vi "BioFeedback14(Small Buckets +Envelope).vi"(7 "Frames Per Second":dbl=30.0, 9 "Start Trial":bool, 11 "End Trial":bool, 12 "Data Directory":path, 13 "File Name":string, 14 "Extension":string="_EMG.txt") -> ()   [LabVIEW 2016]
uses:
  <vilib>/Waveform/WDTOps.llb/WDT Append Waveforms DBL.vi
  <vilib>/Utility/error.llb/DialogType.ctl
  <vilib>/Utility/file.llb/Write Delimited Spreadsheet (string).vi
  <vilib>/Waveform/WDTFileIO.llb/Export Waveforms To Spreadsheet File (1D).vi
  customSubVIs/Control 1.ctl
panel:
  out "FilteredTrialData One Channel":waveform(dbl)(graph)
  out "Raw Trial Data One  Channel":waveform(dbl)(graph)
  out "DisplayMaxTrialsArray":dbl[][](array[numeric])
  out "DisplayMaxArray":dbl[](array[numeric])
  out "EndProcessTic":u32
  out "StartProcessTic":u32
  out "EndRecordTic":u32
  out "startRecordTic":u32
  out "Start UI":timestamp
  out "UI Elapsed Time":u32
  out "End UI":timestamp
  out "End Process":timestamp
  out "Start Process":timestamp
  out "End Record":timestamp
  out "Start Record":timestamp
  out "Process Elapsed Time":u32
  out "Record Elapsed Time":u32
  out "FilteredTrialData":waveform(dbl)[](graph)
  out "FilteredAndRectified":waveform(dbl)[](graph) caption="Filtered and Rectified"
  out "FilteredTrialData":waveform(dbl)[](array[waveform])
  in  "DisplayChannel":dbl
  out "DisplayTrialData":T1
  out "DisplayValueByChannel":dbl[](array[numeric])
  out "DataBufferSize":dbl
  in  "Big Window Length (s)":dbl=0.5
  out "CurrentAvgByChannel":dbl[](array[numeric])
  out "BigBucketBuilder":dbl[][](array[numeric])
  out "Trial Data Column Headers":string[](array[string])
  in  "TrialDataRowHeaders":string[](array[string])=["Wfm1", "Wfm2", "Wfm3", "Wfm4", "Wfm5", "Wfm6", "Wfm7", "Wfm8"]
  out "GetMaxStartTime":timestamp
  in  "SecondsToAcquireMax":dbl=10.0
  in  "NumberOfMaximumsToTake":dbl=3.0
  in  "CurrentMaxIndex":dbl
  out "SignalsMaxArray":dbl[](array[numeric])
  out "SignalMaxTrialsArray":dbl[][](array[numeric])
  in  "%StdDevIndex":dbl=5.0
  in  "Mean%Index":dbl=4.0
  in  "StdDevIndex":dbl=3.0
  in  "MeanIndex":dbl=2.0
  in  "MaxIndex":dbl=1.0
  in  "MinIndex":dbl
  out "Stability Data":dbl[][](array[numeric])
  out "RawTrialData":waveform(dbl)[](array[waveform])
  in  "UI Ampl Error Path":path=path "C:/Users/Tinggroup/Desktop/VRMuscleActivationVisualizer/VRBiofeedback_v2/assets/BiofeedbackAmplitudeError.txt"
  out "DisplayActivation":dbl
  out "Acquiring Max":bool
  in  "resetMax":bool
  in  "startGetMax":bool
  in  "Amplitude Error":dbl
  in  "UI Data Path":path=path "C:/Users/Tinggroup/Desktop/VRMuscleActivationVisualizer/VRBiofeedback_v2/assets/LeftEMGData.txt"
  in  "EMG Input Device\nProduct Type":string="USB-6009"
  out "DisplayBarActivation":dbl(slide) caption="Left" max=1.0 scale=0.0..100.0
  out "NormalizedSignal8":dbl[](graph)
  out "NormalizedSignal7":dbl[](graph)
  out "NormalizedSignal6":dbl[](graph)
  out "NormalizedSignal5":dbl[](graph)
  out "NormalizedSignal4":dbl[](graph)
  out "NormalizedSignal3":dbl[](graph)
  out "NormalizedSignal2":dbl[](graph)
  out "NormalizedSignal1":dbl[](graph)
  out "Raw Trial Data Wfm":waveform(dbl)[](graph)
  in  "UI Percent Path":path=path "C:/Users/Tinggroup/Desktop/VRMuscleActivationVisualizer/VRBiofeedback_v2/assets/BiofeedbackTargetPercentage.txt"
  in  "Target Percentage":dbl=10.0
  out "Trial In Progress":bool
  in  "Lower Cut-Off":dbl=20.0
  in  "Upper Cut-Off":dbl=300.0
  out "raw data":dynamicdata(graph)
  out "DataBufferIndices":dbl[](array[numeric])
  out "SmallBucketSize":dbl
  out "Samples per frame":dbl
  out "Reset Data Acquisition\nAnd UI Updating":bool=TRUE
  in  "Small Window Length (s)":dbl=0.02
  in  "Sample rate (Hz)":dbl=2000.0
  in  "End Program":bool
  # "Data To Be Saved (Not including Max Data)"
  # "Performance Metrics"
  # "Saving Trial Data"
  # "Small Window"
  # "Set Target"
  # "Scale Max"
  # "Filter and Process Parameters"
  # "MVC Scaling Variables"
  # "Start and end recording for max?"
  # "Big Window"
  # "Display Parameters"
  # "Changes are made instantly and cause moving average to reset to zero"
  # "Analyze Stability of Displayed Data (Not Functional)"
  # "Auto Analyze Stability begins calculating stability\nAs soon as dot enters the target zone and stops \nonce the dot leaves the target zone (Not Yet Implemented)"
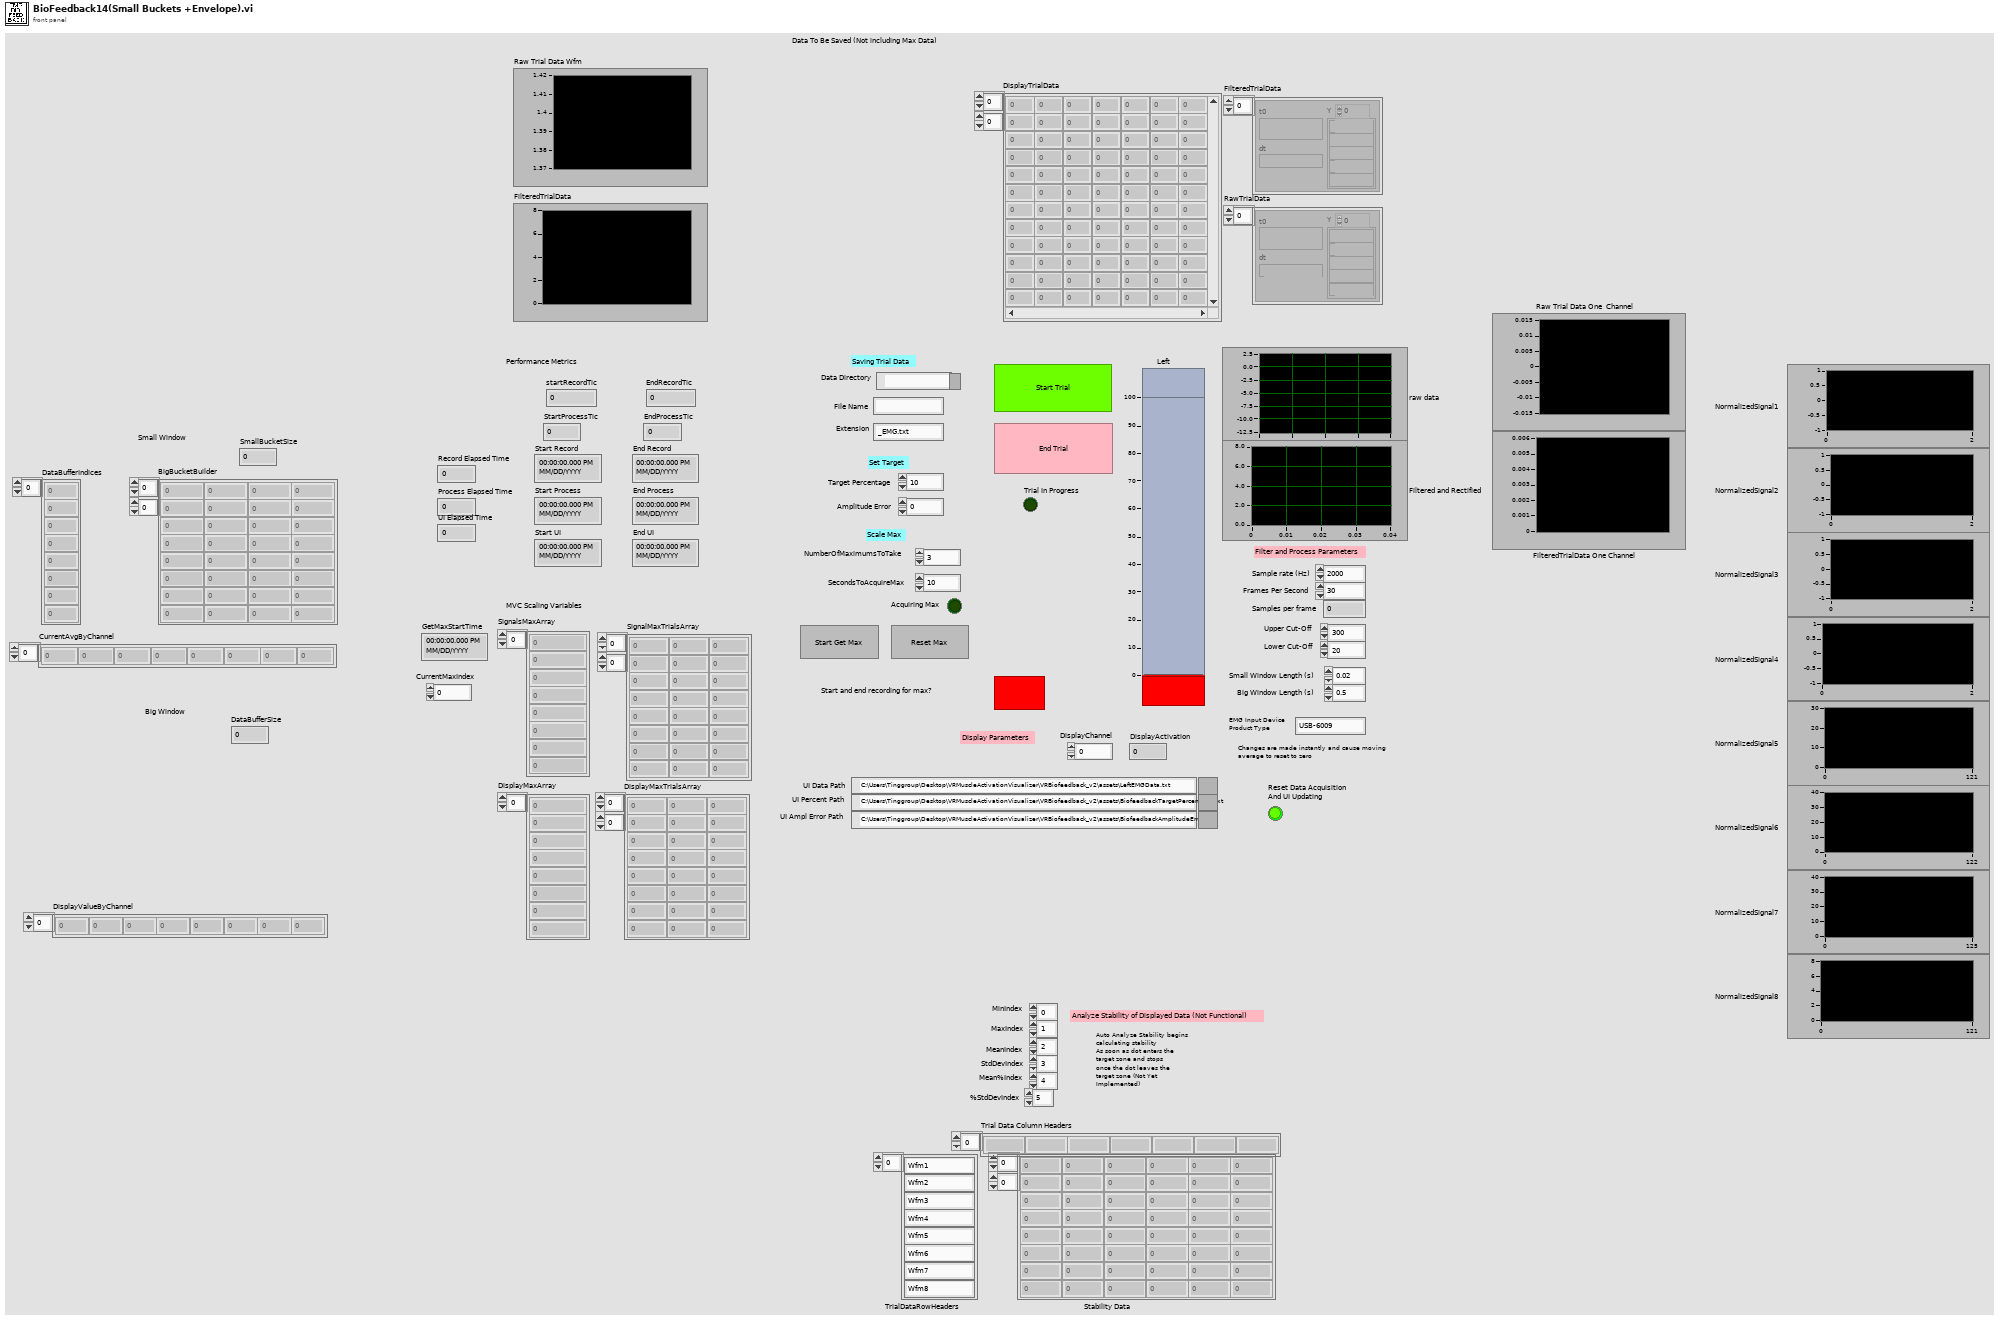
[diagram p1: front panel]
types:
  T1 = typedef "Control 1.ctl" = dbl[][]
  T2 = typedef "DialogType.ctl" = u16
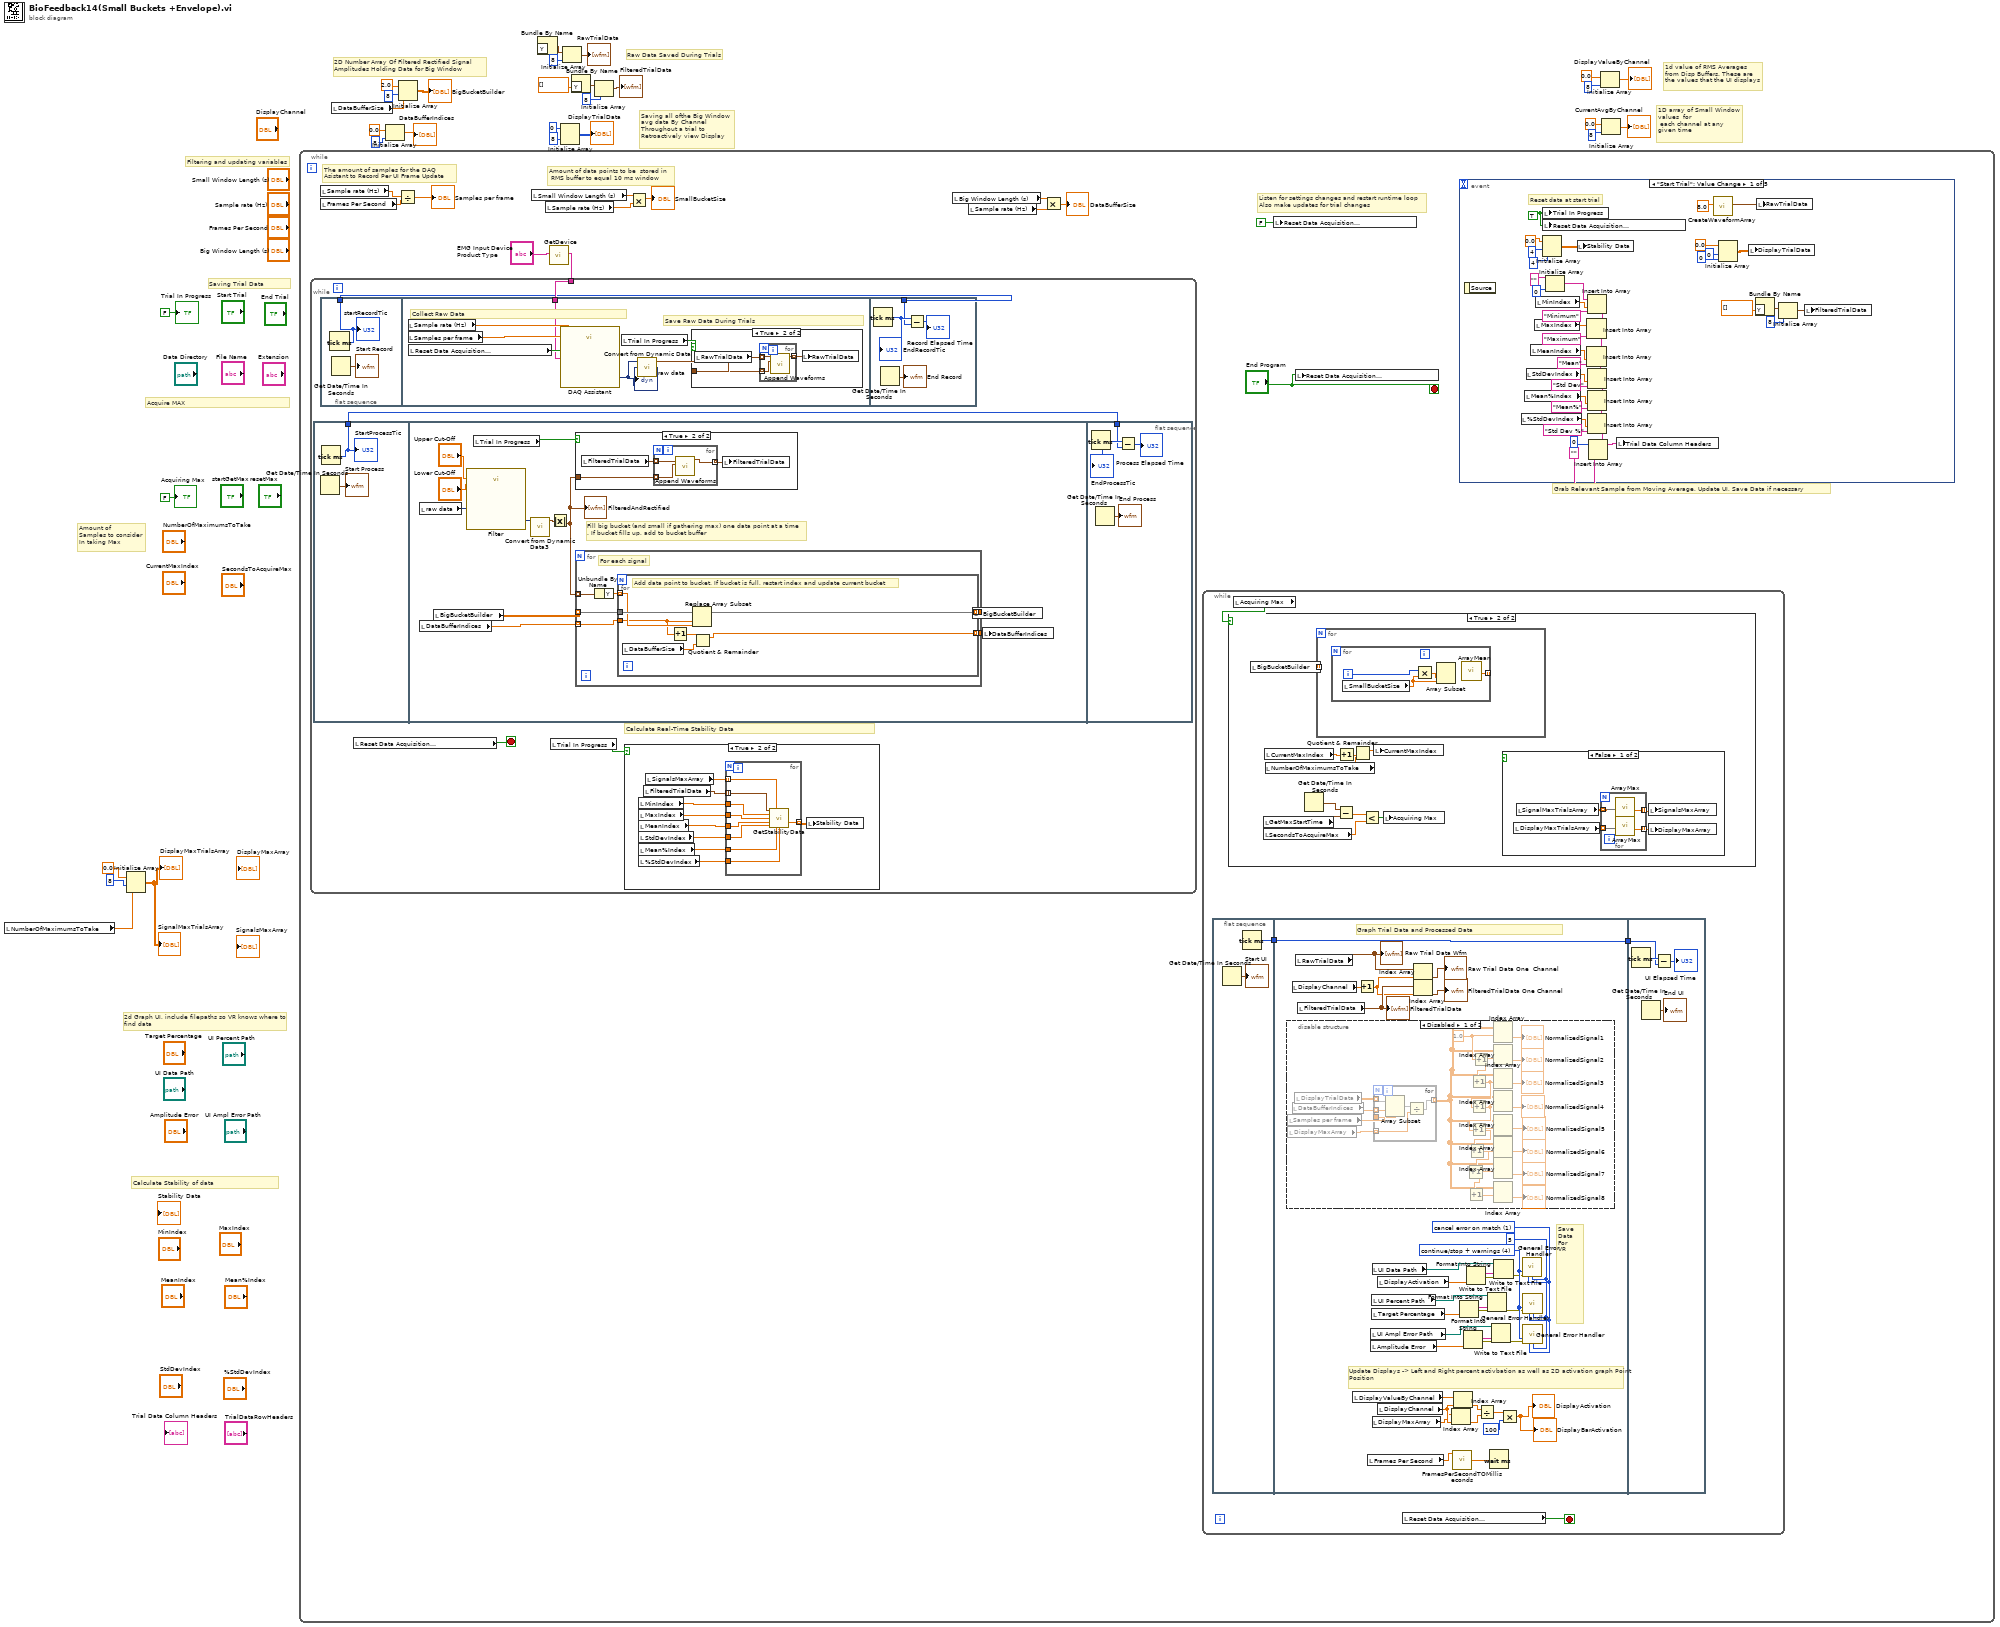
[diagram p0: block diagram]
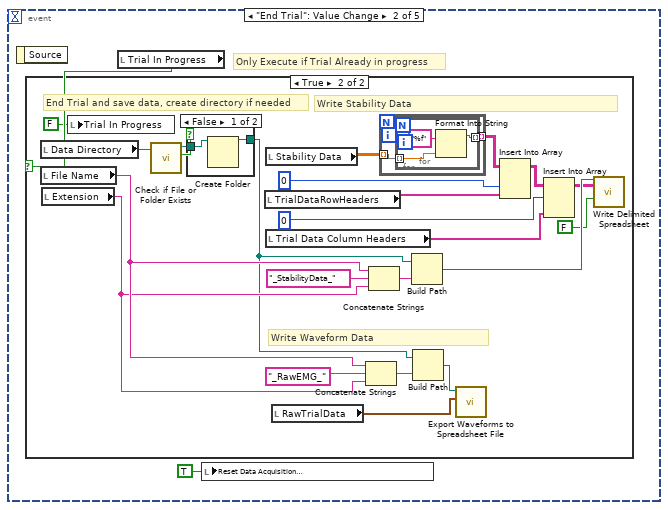
[diagram p5: hidden frame]
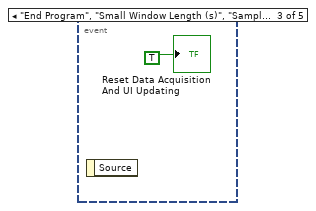
[diagram p8: hidden frame]
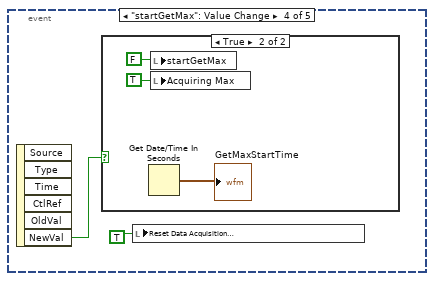
[diagram p9: hidden frame]
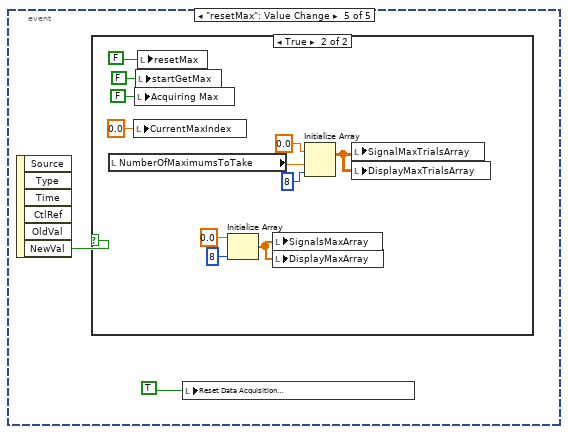
[diagram p11: hidden frame]
diagram:
  # "2D Number Array Of Filtered Rectified Signal Amplitudes Holding Data for Big Window"
  # "Saving all ofthe Big Window \navg data By Channel\nThroughout a trial to \nRetroactively view Display"
  # "1d value of RMS Averages\nfrom Disp Buffers. These are\nthe values that the UI displays"
  # "1D array of Small Window\nvalues  for\n each channel at any\ngiven time"
  # "Raw Data Saved During Trials"
  # "Amount of \nSamples to consider\nIn taking Max"
  # "Calculate Stability of data"
  # "Acquire MAX"
  # "Filtering and updating variables"
  # "Saving Trial Data"
  # "2d Graph UI, include filepaths so VR knows where to find data"
  n1 = local read "NumberOfMaximumsToTake"() -> (w17:dbl)
  n2 = Initialize Array(0.0 ("element"), 8 ("dimension size"), w17) -> (→"SignalMaxTrialsArray" →"DisplayMaxTrialsArray":dbl[][])
  n3 = while {
    stop <- "End Program" stop-if-true
    # "Grab Relevant Sample from Moving Average, Update UI, Save Data if necessary"
    # "Amount of data points to be  stored in\n RMS buffer to equal 10 ms window"
    # "The amount of samples for the DAQ Asistant to Record Per UI Frame Update"
    # "Listen for settings changes and restart runtime loop\nAlso make updates for trial changes"
    n4 = local read "Sample rate (Hz)"() -> (w42:dbl)
    n5 = local read "Frames Per Second"() -> (w41:dbl)
    n6 = Divide(x=w42, y=w41) -> (x/y=→"Samples per frame":dbl)
    n7 = local read "Small Window Length (s)"() -> (w34:dbl)
    n8 = local read "Sample rate (Hz)"() -> (w35:dbl)
    n9 = call "GetDevice.vi"("EMG Input Device\nProduct Type"="EMG Input Device\nProduct Type") -> ("DAQmx Device Name"=w36:tag)  [unwired: 10 in]
    n10 = while {
      tunnel: w36 -> [w232]
      stop <- w230 stop-if-true
      # "Calculate Real-Time Stability Data"
      n11 = flat-sequence {
        tunnel: [w234] -> w229
        tunnel: w229 -> [w266]
        frame #0 {
          n12 = Get Date/Time In Seconds() -> (seconds since 1Jan1904=→"Start Process":timestamp)
          n13 = Tick Count (ms)() -> (millisecond timer value=w234:u32)
          "StartProcessTic" <- w234
        }
        frame #1 {
          # "Fill big bucket (and small if gathering max) one data point at a time\n. If bucket fills up, add to bucket buffer"
          n14 = local read "raw data"() -> (w245:dynamicdata)
          n15 = local read "DataBufferIndices"() -> (w237:dbl[])
          n16 = local read "BigBucketBuilder"() -> (w238:dbl[][])
          n17 = call "Filter"("Lower Cut-Off"="Lower Cut-Off", "Upper Cut-Off"="Upper Cut-Off", "Signal"=w245) -> ("Filtered Signal"=w244:dynamicdata)  [unwired: 7 in, 1 out]
          n18 = local read "Trial In Progress"() -> (w240:bool)
          n19 = call "Convert from Dynamic Data3"("Dynamic Data Type"=w244) -> ("Array of Waveform"=w243:waveform(dbl)[])  [unwired: 3 in]
          n20 = Absolute Value(x=w243) -> (abs(x)=w239:waveform(dbl)[])
          "FilteredAndRectified" <- w239
          n21 = case shown="True" w240 {
            tunnel: w239 -> [_ w260]
            frame False {
            }
            frame True {
              n22 = local read "FilteredTrialData"() -> (w261:waveform(dbl)[])
              n23 = for {
                tunnel: w261 -> [w264] mode=indexing
                tunnel: w260 -> [w263] mode=indexing
                tunnel: [w262] -> w259 mode=indexing
                n24 = call-poly <vilib>:"Append Waveforms.vi"("waveform B"=w263, "waveform A"=w264) -> ("waveform out"=w262:waveform(dbl))  [unwired: 8 in, 1 out]
              }
              n25 = local write "FilteredTrialData"(w259) -> ()
            }
          }
          n26 = for {
            tunnel: w239 -> [w251] mode=indexing
            tunnel: w238 -> [w249] mode=indexing
            tunnel: w237 -> [w248] mode=indexing
            tunnel: [w247] -> w236
            tunnel: [w246] -> w235
            # "For each signal"
            n27 = Unbundle By Name(w251) -> ("Y"=w250:dbl[])
            n28 = for {
              tunnel: w250 -> [w257] mode=indexing
              tunnel: w249 -> [w258]
              tunnel: w248 -> [w256]
              tunnel: [w253] -> w247 mode=indexing
              tunnel: [w252] -> w246 mode=indexing
              # "Add data point to bucket. If bucket is full, restart index and update current bucket"
              n29 = local read "DataBufferSize"() -> (w254:dbl)
              n30 = Increment(x=w256) -> (x+1=w255:dbl)
              n31 = Replace Array Subset(array=w258, new element=w257, index=w256) -> (w253:dbl[])
              n32 = Quotient & Remainder(x=w255, y=w254) -> (x-y*floor(x/y)=w252:dbl)  [unwired: 1 out]
            }
          }
          n33 = local write "BigBucketBuilder"(w236) -> ()
          n34 = local write "DataBufferIndices"(w235) -> ()
        }
        frame #2 {
          n35 = Tick Count (ms)() -> (millisecond timer value=w267:u32)
          "EndProcessTic" <- w267
          n36 = Get Date/Time In Seconds() -> (seconds since 1Jan1904=→"End Process":timestamp)
          n37 = Subtract(x=w267, y=w266) -> (x-y=→"Process Elapsed Time":u32)
        }
      }
      n38 = flat-sequence {
        tunnel: [w270] -> w228
        tunnel: w232 -> [w271]
        tunnel: w228 -> [w284]
        frame #0 {
          n39 = Tick Count (ms)() -> (millisecond timer value=w270:u32)
          "startRecordTic" <- w270
          n40 = Get Date/Time In Seconds() -> (seconds since 1Jan1904=→"Start Record":timestamp)
        }
        frame #1 {
          # "Save Raw Data During Trials"
          # "Collect Raw Data"
          n41 = local read "Sample rate (Hz)"() -> (w274:dbl)
          n42 = local read "Samples per frame"() -> (w273:dbl)
          n43 = local read "Reset Data Acquisition\nAnd UI Updating"() -> (w272:bool)
          n44 = call "DAQ Assistant"("rate"=w274, "number of samples"=w273, "stop (T)"=w272, "device name"=w271) -> ("data"=w276:dynamicdata)  [unwired: 13 in, 2 out]
          "raw data" <- w276
          n45 = local read "Trial In Progress"() -> (w277:bool)
          n46 = call "Convert from Dynamic Data"("Dynamic Data Type"=w276) -> ("Array of Waveform"=w275:waveform(dbl)[])  [unwired: 3 in]
          n47 = case shown="True" w277 {
            tunnel: w275 -> [_ w280]
            frame False {
            }
            frame True {
              n48 = local read "RawTrialData"() -> (w279:waveform(dbl)[])
              n49 = for {
                tunnel: w280 -> [w282] mode=indexing
                tunnel: w279 -> [w283] mode=indexing
                tunnel: [w281] -> w278 mode=indexing
                n50 = call-poly <vilib>:"Append Waveforms.vi"("waveform B"=w282, "waveform A"=w283) -> ("waveform out"=w281:waveform(dbl))  [unwired: 8 in, 1 out]
              }
              n51 = local write "RawTrialData"(w278) -> ()
            }
          }
        }
        frame #2 {
          n52 = Tick Count (ms)() -> (millisecond timer value=w285:u32)
          "EndRecordTic" <- w285
          n53 = Get Date/Time In Seconds() -> (seconds since 1Jan1904=→"End Record":timestamp)
          n54 = Subtract(x=w285, y=w284) -> (x-y=→"Record Elapsed Time":u32)
        }
      }
      n55 = local read "Reset Data Acquisition\nAnd UI Updating"() -> (w230:bool)
      n56 = local read "Trial In Progress"() -> (w231:bool)
      n57 = case shown="True" w231 {
        frame False {
        }
        frame True {
          n58 = local read "MinIndex"() -> (w295:dbl)
          n59 = local read "MaxIndex"() -> (w294:dbl)
          n60 = local read "MeanIndex"() -> (w293:dbl)
          n61 = local read "StdDevIndex"() -> (w292:dbl)
          n62 = local read "Mean%Index"() -> (w291:dbl)
          n63 = local read "%StdDevIndex"() -> (w290:dbl)
          n64 = local read "FilteredTrialData"() -> (w296:waveform(dbl)[])
          n65 = local read "SignalsMaxArray"() -> (w288:dbl[])
          n66 = for {
            tunnel: w296 -> [w297] mode=indexing
            tunnel: [w298] -> w289 mode=indexing
            tunnel: w295 -> [w305]
            tunnel: w294 -> [w304]
            tunnel: w293 -> [w303]
            tunnel: w292 -> [w302]
            tunnel: w291 -> [w301]
            tunnel: w290 -> [w300]
            tunnel: w288 -> [w299] mode=indexing
            n67 = call "GetStabilityData.vi"("ProvidedData"=w297, "ScaleMax"=w299, "MinIndex"=w305, "MaxIndex"=w304, "MeanIndex"=w303, "StdDevIndex"=w302, "Mean%Index"=w301, "%StdDevIndex"=w300) -> ("ReturnData"=w298:dbl[])  [unwired: 7 in]
          }
          n68 = local write "Stability Data"(w289) -> ()
        }
      }
    }
    n69 = Multiply(x=w34, y=w35) -> (x*y=→"SmallBucketSize":dbl)
    n70 = local read "Big Window Length (s)"() -> (w32:dbl)
    n71 = local read "Sample rate (Hz)"() -> (w30:dbl)
    n72 = Multiply(x=w32, y=w30) -> (x*y=→"DataBufferSize":dbl)
    n73 = while {
      stop <- w44 stop-if-true
      n74 = flat-sequence {
        tunnel: [w70] -> w46
        tunnel: [w105] -> w45
        tunnel: w46 -> [w105]
        tunnel: w45 -> [w133]
        frame #0 {
          n75 = Get Date/Time In Seconds() -> (seconds since 1Jan1904=→"Start UI":timestamp)
          n76 = Tick Count (ms)() -> (millisecond timer value=w70:u32)
        }
        frame #1 {
          w100 = T2 4 items=["no dialog", "OK message", "continue or stop message", "OK message + warnings", "continue/stop + warnings"] ("type of dialog (OK msg:1)")
          w101 = 1 items=["no exception", "cancel error on match", "set error on match"] ("[exception action] (none:0)")
          w102 = 5 ("[exception code]")
          # "Graph Trial Data and Processed Data"
          # "Update Displays -> Left and Right percent activbation as well as 2D activation graph Point Position"
          # "Save\nData\nFor\nVR"
          n77 = disable-structure shown="Disabled" {
            frame Disabled {
              w126 = 1.0 ("x")
              n78 = local read "Samples per frame"() -> (w107:dbl)
              n79 = local read "DisplayMaxArray"() -> (w106:dbl[])
              n80 = local read "DataBufferIndices"() -> (w108:dbl[])
              n81 = local read "DisplayTrialData"() -> (w109:T1)
              n82 = for {
                tunnel: w109 -> [w131] mode=indexing
                tunnel: w106 -> [w127] mode=indexing
                tunnel: [w132] -> w110 mode=indexing
                tunnel: w108 -> [w130] mode=indexing
                tunnel: w107 -> [w129]
                n83 = Array Subset(array=w131, index=w130, length=w129) -> (w128:dbl[])
                n84 = Divide(x=w128, y=w127) -> (x/y=w132:dbl[])
              }
              n85 = Increment(x=w126) -> (x+1=w125:dbl)
              n86 = Increment(x=w125) -> (x+1=w124:dbl)
              n87 = Increment(x=w124) -> (x+1=w123:dbl)
              n88 = Increment(x=w123) -> (x+1=w122:dbl)
              n89 = Increment(x=w122) -> (x+1=w121:dbl)
              n90 = Increment(x=w121) -> (x+1=w120:dbl)
              n91 = Increment(x=w120) -> (x+1=w119:dbl)
              n92 = Index Array(array=w110, index (row)=w126) -> (element=→"NormalizedSignal1":dbl[])  [unwired: 1 in]
              n93 = Index Array(array=w110, index (row)=w125) -> (element=→"NormalizedSignal2":dbl[])  [unwired: 1 in]
              n94 = Index Array(array=w110, index (row)=w124) -> (element=→"NormalizedSignal3":dbl[])  [unwired: 1 in]
              n95 = Index Array(array=w110, index (row)=w123) -> (element=→"NormalizedSignal4":dbl[])  [unwired: 1 in]
              n96 = Index Array(array=w110, index (row)=w122) -> (element=→"NormalizedSignal5":dbl[])  [unwired: 1 in]
              n97 = Index Array(array=w110, index (row)=w121) -> (element=→"NormalizedSignal6":dbl[])  [unwired: 1 in]
              n98 = Index Array(array=w110, index (row)=w120) -> (element=→"NormalizedSignal7":dbl[])  [unwired: 1 in]
              n99 = Index Array(array=w110, index (row)=w119) -> (element=→"NormalizedSignal8":dbl[])  [unwired: 1 in]
            }
            frame Enabled {
            }
          }
          n100 = local read "DisplayChannel"() -> (w76:dbl)
          n101 = local read "RawTrialData"() -> (w75:waveform(dbl)[])
          "Raw Trial Data Wfm" <- w75
          n102 = local read "FilteredTrialData"() -> (w74:waveform(dbl)[])
          "FilteredTrialData" <- w74
          n103 = local read "DisplayValueByChannel"() -> (w104:dbl[])
          n104 = Increment(x=w76) -> (x+1=w73:dbl)
          n105 = local read "Frames Per Second"() -> (w82:dbl)
          n106 = local read "UI Ampl Error Path"() -> (w99:path)
          n107 = local read "Amplitude Error"() -> (w98:dbl)
          n108 = local read "UI Percent Path"() -> (w91:path)
          n109 = local read "Target Percentage"() -> (w92:dbl)
          n110 = local read "UI Data Path"() -> (w85:path)
          n111 = local read "DisplayMaxArray"() -> (w77:dbl[])
          n112 = local read "DisplayActivation"() -> (w87:dbl)
          n113 = local read "DisplayChannel"() -> (w78:dbl)
          n114 = Index Array(array=w75, index=w73) -> (element=→"Raw Trial Data One  Channel":waveform(dbl))
          n115 = Index Array(array=w74, index=w73) -> (element=→"FilteredTrialData One Channel":waveform(dbl))
          n116 = Index Array(array=w77, index=w78) -> (element=w79:dbl)
          n117 = call "FramesPerSecondTOMilliseconds.vi"("Thermometer\nFps"=w82) -> ("x*y"=w103:dbl)  [unwired: 10 in]
          n118 = Index Array(array=w104, index=w78) -> (element=w81:dbl)
          n119 = Format Into String(w92) -> (resulting string=w90:string, error out=w89:errorcluster)  [unwired: 3 in]
          n120 = Format Into String(w98) -> (resulting string=w97:string, error out=w96:errorcluster)  [unwired: 3 in]
          n121 = Format Into String(w87) -> (resulting string=w86:string, error out=w84:errorcluster)  [unwired: 3 in]
          n122 = Divide(x=w81, y=w79) -> (x/y=w94:dbl)
          n123 = Write to Text File(file (use dialog)=w91, text=w90, error in=w89) -> (error out=w88:errorcluster)  [unwired: 1 in, 2 out]
          n124 = Wait (ms)(milliseconds to wait=w103) -> ()  [unwired: 1 out]
          n125 = Write to Text File(file (use dialog)=w99, text=w97, error in=w96) -> (error out=w95:errorcluster)  [unwired: 1 in, 2 out]
          n126 = Write to Text File(file (use dialog)=w85, text=w86, error in=w84) -> (error out=w83:errorcluster)  [unwired: 1 in, 2 out]
          n127 = Multiply(x=w94, y=100) -> (x*y=→"DisplayBarActivation" →"DisplayActivation":dbl)
          n128 = call <vilib>:"General Error Handler.vi"("type of dialog (OK msg:1)"=w100, "error in (no error)"=w83, "[exception action] (none:0)"=w101, "[exception code]"=w102) -> ()  [unwired: 7 in, 5 out]
          n129 = call <vilib>:"General Error Handler.vi"("type of dialog (OK msg:1)"=w100, "error in (no error)"=w88, "[exception action] (none:0)"=w101, "[exception code]"=w102) -> ()  [unwired: 7 in, 5 out]
          n130 = call <vilib>:"General Error Handler.vi"("type of dialog (OK msg:1)"=w100, "error in (no error)"=w95, "[exception action] (none:0)"=w101, "[exception code]"=w102) -> ()  [unwired: 7 in, 5 out]
        }
        frame #2 {
          n131 = Tick Count (ms)() -> (millisecond timer value=w134:u32)
          n132 = Get Date/Time In Seconds() -> (seconds since 1Jan1904=→"End UI":timestamp)
          n133 = Subtract(x=w134, y=w133) -> (x-y=→"UI Elapsed Time":u32)
        }
      }
      n134 = local read "Acquiring Max"() -> (w43:bool)
      n135 = case shown="True" w43 {
        frame False {
        }
        frame True {
          n136 = local read "BigBucketBuilder"() -> (w47:dbl[][])
          n137 = local read "GetMaxStartTime"() -> (w56:timestamp)
          n138 = local read "SecondsToAcquireMax"() -> (w53:dbl)
          n139 = local read "CurrentMaxIndex"() -> (w51:dbl)
          n140 = local read "NumberOfMaximumsToTake"() -> (w49:dbl)
          n141 = Get Date/Time In Seconds() -> (seconds since 1Jan1904=w55:timestamp)
          n142 = for {
            tunnel: w47 -> [_] mode=indexing
            n143 = for {
              tunnel: [w57] -> _ mode=indexing
              i -> [w58]
              n144 = local read "SmallBucketSize"() -> (w59:dbl)
              n145 = Multiply(x=w58, y=w59) -> (x*y=w60:dbl)
              n146 = Array Subset(index=w60, length=w59) -> ()  [unwired: 1 in, 1 out]
              n147 = call "ArrayMean.vi"() -> ("Mean"=w57:dbl)  [unwired: 11 in]
            }
          }
          n148 = Subtract(x=w55, y=w56) -> (x-y=w54:dbl)
          n149 = Increment(x=w51) -> (x+1=w50:dbl)
          n150 = Quotient & Remainder(x=w50, y=w49) -> (x-y*floor(x/y)=w48:dbl)  [unwired: 1 out]
          n151 = Less?(x=w54, y=w53) -> (x < y?=w52:bool)
          n152 = local write "CurrentMaxIndex"(w48) -> ()
          n153 = local write "Acquiring Max"(w52) -> ()
          n154 = case shown="False" {
            selector: _ -> [_ _]
            frame False {
              n155 = local read "DisplayMaxTrialsArray"() -> (w62:dbl[][])
              n156 = local read "SignalMaxTrialsArray"() -> (w64:dbl[][])
              n157 = for {
                tunnel: w64 -> [w68] mode=indexing
                tunnel: [w67] -> w63 mode=indexing
                tunnel: w62 -> [w66] mode=indexing
                tunnel: [w65] -> w61 mode=indexing
                n158 = call "ArrayMax.vi"("Array"=w66) -> ("max"=w65:dbl)  [unwired: 10 in]
                n159 = call "ArrayMax.vi"("Array"=w68) -> ("max"=w67:dbl)  [unwired: 10 in]
              }
              n160 = local write "SignalsMaxArray"(w63) -> ()
              n161 = local write "DisplayMaxArray"(w61) -> ()
            }
            frame True {
            }
          }
        }
      }
      n162 = local read "Reset Data Acquisition\nAnd UI Updating"() -> (w44:bool)
    }
    n163 = local write "Reset Data Acquisition\nAnd UI Updating"(FALSE) -> ()
    n164 = local write "Reset Data Acquisition\nAnd UI Updating"("End Program") -> ()
    n165 = event shown="[0] \"Start Trial\": Value Change" {
      selector: _ -> [_ _ _ _ _]
      dyn-events: _ -> [_ _ _ _ _]
      timeout: _ -> [_ _ _ _ _]
      event "Start Trial": Value Change {
        w175 = TRUE ("Trial In Progress")
        # "Reset data at start trial"
        n166 = event-data() -> ()  [unwired: 1 in, 1 out]
        n167 = local read "%StdDevIndex"() -> (w151:dbl)
        n168 = local read "Mean%Index"() -> (w152:dbl)
        n169 = local read "StdDevIndex"() -> (w156:dbl)
        n170 = local read "MeanIndex"() -> (w160:dbl)
        n171 = local read "MaxIndex"() -> (w163:dbl)
        n172 = local read "MinIndex"() -> (w165:dbl)
        n173 = Initialize Array(0.0 ("element"), 4 ("dimension size"), 4 ("dimension size")) -> (w169:dbl[][])
        n174 = local write "Trial In Progress"(w175) -> ()
        n175 = local write "Reset Data Acquisition\nAnd UI Updating"(w175) -> ()
        n176 = Initialize Array("", 0 ("dimension size")) -> (w164:string[])
        n177 = local write "Stability Data"(w169) -> ()
        n178 = Insert Into Array(array=w164, index=w165, new element="Minimum" ("new element/subarray")) -> (w161:string[])
        n179 = Insert Into Array(array=w161, index=w163, new element="Maximum" ("new element/subarray")) -> (w158:string[])
        n180 = Insert Into Array(array=w158, index=w160, new element="Mean" ("new element/subarray")) -> (w155:string[])
        n181 = Insert Into Array(array=w155, index=w156, new element="Std Dev" ("new element/subarray")) -> (w153:string[])
        n182 = Insert Into Array(array=w153, index=w152, new element="Mean%" ("new element/subarray")) -> (w149:string[])
        n183 = Insert Into Array(array=w149, index=w151, new element="Std Dev %" ("new element/subarray")) -> (w146:string[])
        n184 = Insert Into Array(array=w146, index=0, new element="" ("new element/subarray")) -> (w147:string[])
        n185 = local write "Trial Data Column Headers"(w147) -> ()
        n186 = call "CreateWaveformArray.vi"("bufferSize"=8.0) -> ("initialized array"=w174:waveform(dbl)[])  [unwired: 5 in, 1 out]
        n187 = Initialize Array(0.0 ("element"), 0 ("dimension size"), 0 ("dimension size")) -> (w141:dbl[][])
        n188 = local write "DisplayTrialData"(w141) -> ()
        n189 = Bundle By Name("Y"=dbl[] []) -> (w140:waveform(dbl))  [unwired: 1 in]
        n190 = local write "RawTrialData"(w174) -> ()
        n191 = Initialize Array(w140, 8 ("dimension size")) -> (w137:waveform(dbl)[])
        n192 = local write "FilteredTrialData"(w137) -> ()
      }
      event "End Trial": Value Change {
        # "Only Execute if Trial Already in progress"
        n193 = event-data() -> ()  [unwired: 1 in, 1 out]
        n194 = local read "Trial In Progress"() -> (w177:bool)
        n195 = case shown="True" w177 {
          frame False {
          }
          frame True {
            # "Write Waveform Data"
            # "Write Stability Data"
            # "End Trial and save data, create directory if needed"
            n196 = local read "Data Directory"() -> (w197:path)
            n197 = local read "File Name"() -> (w183:string)
            n198 = local read "Extension"() -> (w182:string)
            n199 = local write "Trial In Progress"(FALSE ("Trial In Progress")) -> ()
            n200 = call <vilib>:"Check if File or Folder Exists.vi"("path"=w197) -> ("file or folder exists?"=w199:bool, "dup path"=w198:path)  [unwired: 8 in, 1 out]
            n201 = case shown="False" w199 {
              tunnel: [w206 w208] -> w181
              tunnel: w198 -> [w207 w208]
              frame False {
                n202 = Create Folder(path (use dialog)=w207) -> (created path=w206:path)  [unwired: 2 in, 2 out]
              }
              frame True {
              }
            }
            n203 = local read "TrialDataRowHeaders"() -> (w192:string[])
            n204 = local read "Stability Data"() -> (w189:dbl[][])
            n205 = local read "Trial Data Column Headers"() -> (w193:string[])
            n206 = local read "RawTrialData"() -> (w179:waveform(dbl)[])
            n207 = Concatenate Strings(w183, "_RawEMG_" ("string"), w182) -> (w180:string)
            n208 = Concatenate Strings(w183, "_StabilityData_" ("string"), w182) -> (w185:string)
            n209 = for {
              tunnel: w189 -> [w202] mode=indexing
              tunnel: [w201] -> w187 mode=indexing
              n210 = for {
                tunnel: w202 -> [w204] mode=indexing
                tunnel: [w203] -> w201 mode=indexing
                n211 = Format Into String(format string="%f", w204) -> (resulting string=w203:string)  [unwired: 2 in, 1 out]
              }
            }
            n212 = Build Path(base path=w181, name or relative path=w185) -> (appended path=w195:path)
            n213 = Build Path(base path=w181, name or relative path=w180) -> (appended path=w178:path)
            n214 = call-poly <vilib>:"Export Waveforms to Spreadsheet File.vi"("waveforms"=w179, "file path (dialog if empty)"=w178) -> ()  [unwired: 8 in, 2 out]
            n215 = Insert Into Array(array=w187, index (col)=0 ("index (row)"), new element=w192) -> (w196:string[][])  [unwired: 1 in]
            n216 = Insert Into Array(array=w196, index (row)=0 ("index (col)"), new element=w193) -> (w188:string[][])  [unwired: 1 in]
            n217 = call-poly <vilib>:"Write Delimited Spreadsheet.vi"("file path (dialog if empty)"=w195, "2D data"=w188, "append to file? (new file:F)"=FALSE) -> ()  [unwired: 11 in, 2 out]
          }
        }
        n218 = local write "Reset Data Acquisition\nAnd UI Updating"(TRUE ("Reset Data Acquisition\nAnd UI Updating")) -> ()
      }
      event "End Program", "Small Window Length (s)", "Sample rate (Hz)", "Frames Per Second": Value Change {
        n219 = event-data() -> ()  [unwired: 1 in, 1 out]
        "Reset Data Acquisition\nAnd UI Updating" <- TRUE
      }
      event "startGetMax": Value Change {
        n220 = event-data() -> ("NewVal"=w211:bool)  [unwired: 1 in, 5 out]
        n221 = case shown="True" w211 {
          frame False {
          }
          frame True {
            n222 = Get Date/Time In Seconds() -> (seconds since 1Jan1904=→"GetMaxStartTime":timestamp)
            n223 = local write "startGetMax"(FALSE) -> ()
            n224 = local write "Acquiring Max"(TRUE ("Acquiring Max")) -> ()
          }
        }
        n225 = local write "Reset Data Acquisition\nAnd UI Updating"(TRUE ("Reset Data Acquisition\nAnd UI Updating")) -> ()
      }
      event "resetMax": Value Change {
        n226 = event-data() -> ("NewVal"=w216:bool)  [unwired: 1 in, 5 out]
        n227 = case shown="True" w216 {
          frame False {
          }
          frame True {
            n228 = local read "NumberOfMaximumsToTake"() -> (w223:dbl)
            n229 = local write "CurrentMaxIndex"(0.0 ("CurrentMaxIndex")) -> ()
            n230 = local write "Acquiring Max"(FALSE ("Acquiring Max")) -> ()
            n231 = local write "startGetMax"(FALSE ("startGetMax")) -> ()
            n232 = local write "resetMax"(FALSE ("endGetMax")) -> ()
            n233 = Initialize Array(0.0 ("element"), 8 ("dimension size")) -> (w218:dbl[])
            n234 = local write "SignalsMaxArray"(w218) -> ()
            n235 = local write "DisplayMaxArray"(w218) -> ()
            n236 = Initialize Array(0.0 ("element"), w223, 8 ("dimension size")) -> (w217:dbl[][])
            n237 = local write "SignalMaxTrialsArray"(w217) -> ()
            n238 = local write "DisplayMaxTrialsArray"(w217) -> ()
          }
        }
        n239 = local write "Reset Data Acquisition\nAnd UI Updating"(TRUE ("Reset Data Acquisition\nAnd UI Updating")) -> ()
      }
    }
  }
  n240 = local read "DataBufferSize"() -> (w16:dbl)
  n241 = Initialize Array(0.0 ("element"), 8 ("dimension size")) -> (→"DataBufferIndices":dbl[])
  n242 = Initialize Array(2.0 ("element"), 8 ("dimension size"), w16) -> (→"BigBucketBuilder":dbl[][])
  n243 = Bundle By Name() -> (w10:waveform(dbl))  [unwired: 2 in]
  n244 = Initialize Array(0, 8 ("dimension size")) -> (→"DisplayTrialData":i32[][])  [unwired: 1 in]
  n245 = Initialize Array(w10, 8 ("dimension size")) -> (→"RawTrialData":waveform(dbl)[])
  n246 = Bundle By Name("Y"=dbl[] []) -> (w2:waveform(dbl))  [unwired: 1 in]
  n247 = Initialize Array(w2, 8 ("dimension size")) -> (→"FilteredTrialData":waveform(dbl)[])
  n248 = Initialize Array(0.0 ("element"), 8 ("dimension size")) -> (→"DisplayValueByChannel":dbl[])
  n249 = Initialize Array(0.0 ("element"), 8 ("dimension size")) -> (→"CurrentAvgByChannel":dbl[])
  "Trial In Progress" <- FALSE ("Trial In Progress")
  "Acquiring Max" <- FALSE ("Acquiring Max")
